vi "edit.vi"(8 "error in (no error)":errorcluster, 11 "BaseSetting in":refnum<class "ProcessSettings.lvclass">) -> (0 "error out":errorcluster, 2 "cancelIsTrue out":bool, 3 "BaseSetting out":refnum<class "ProcessSettings.lvclass">)   [LabVIEW 2016, in "Settings.lvlib" / "ProcessSettings.lvclass"]
uses:
  ProcessSettings.lvclass
  home/andres/ct_cmpuserevents/ComponentTemplateCore/Settings/Settings/Setting.lvclass
  ConfigurationTC/ConfigurationTypedefs/Base/SettingAliases.ctl
  ConfigurationTC/ConfigurationTypedefs/Base/SettingAlias.ctl
  ConfigurationTC/ConfigurationTypedefs/Base/RecommendedSettings.ctl
  ConfigurationTC/ConfigurationTypedefs/Base/HeartbeatConfig.ctl
  ConfigurationTC/ConfigurationTypedefs/Base/SALVisSettings.ctl
  MiddlewareSALThisComponent/ProgrammaticInitialization/evntsToSubscribeView.ctl
  MiddlewareSALThisComponent/ProgrammaticInitialization/tlmtryToSubscribeView.ctl
  MiddlewareSALThisComponent/ProgrammaticInitialization/cmdsToSubscribeDL.ctl
  Settings/Setting.lvclass/Setting.ctl
  <vilib>/Utility/xml.llb/Write to XML File(string).vi
  Settings/Setting.lvclass
  ConfigurationTC/ConfigurationTypedefs/ConfigurationTypedefs.lvlib
  MiddlewareSALThisComponent/ProgrammaticInitialization/ProgrammaticInitialization.lvclass
panel:
  in  "SettingTab":T1(tab)
  in  "Aliases":T2
  in  "GenericSALDefinitions":T4={"Subsystem"="EXA", "SAL Vis Path"=path "/home/andres/ts_cbp/ts_sallv_calibrationcbp/VIs", "Events"=["RejectedCommand", "SummaryState", "LoopTimeOutOfRange", "InternalCommand", "Heartbeat", "ErrorCode", "DetailedState", "AppliedSettingsMatchStart", "SettingVersions"], "Telemetry"=["Timestamp", "LoopTimems"], "Commands"=["Start", "Standby", "Enable", "Disable", "ExitControl"]}
  in  "RecommendedSettings":T8
  in  "heartbeatConfig":T9={"Heartbeat Interval (s)"=1.0, "Heartbeat Timeout (s)"=5.0} {"Heartbeat Timeout (s)" min=0.5 max=60.0 step=0.1 format="%.1f"; "Heartbeat Interval (s)" min=0.1 max=10.0 step=0.1 format="%.1f"}
  in  "cancelIsTrue":bool
  out "String":string
  in  "saveIsTrue":bool
  in  "Listbox":i32(listbox)
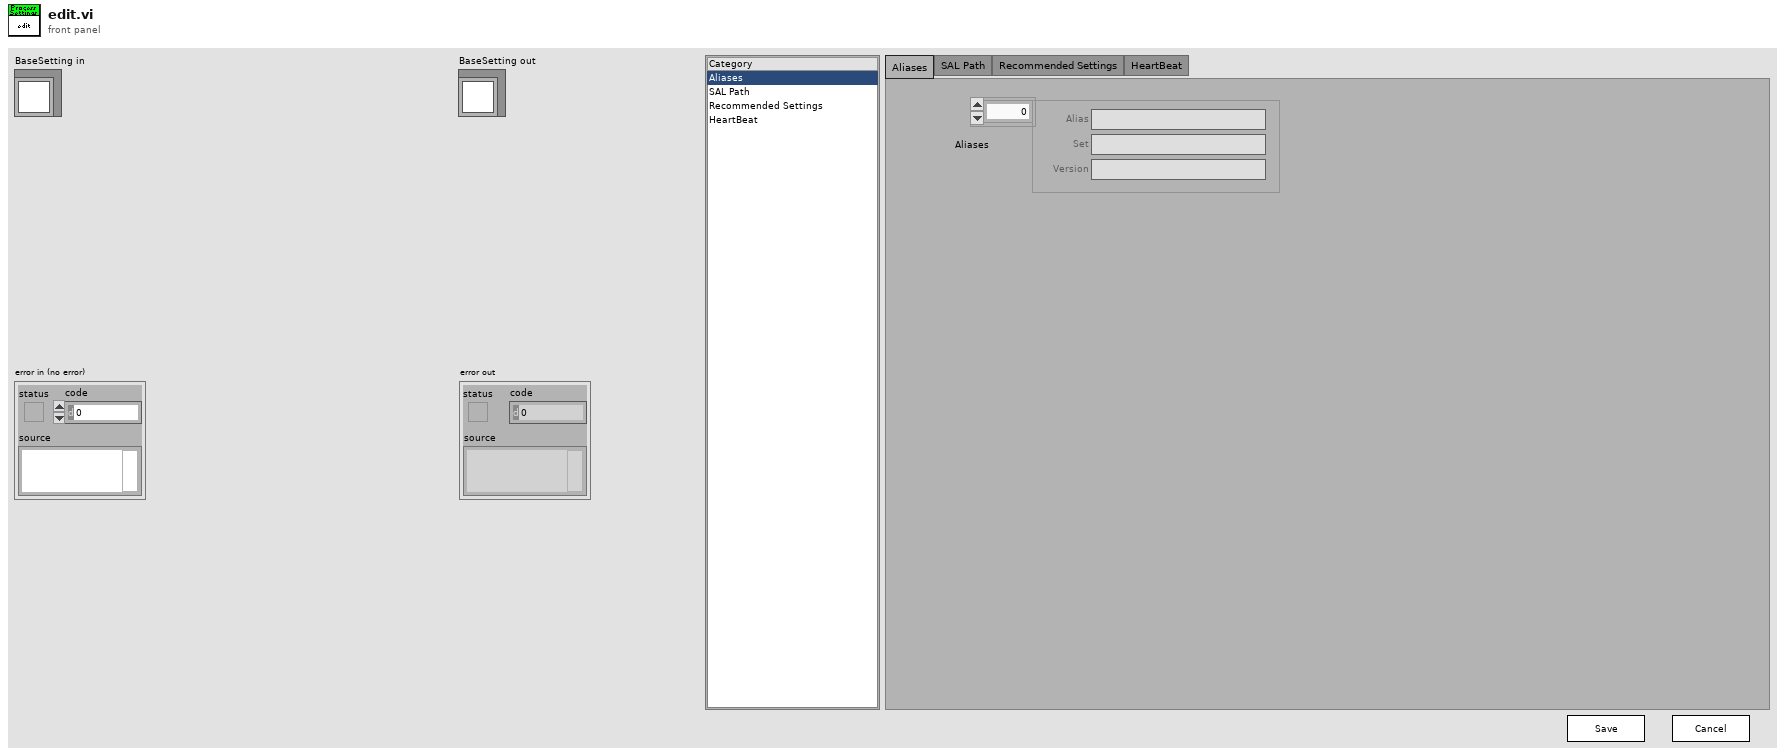
[diagram p1: front panel]
types:
  T1 = enum32{"Aliases", "SAL Path", "Recommended Settings", "HeartBeat"}
  T2 = typedef "ConfigurationTypedefs.lvlib/SettingAliases.ctl" = cluster{"Aliases":T3[]}
  T3 = typedef "ConfigurationTypedefs.lvlib/SettingAlias.ctl" = cluster{"Alias":string, "Set":string, "Version":string}
  T4 = typedef "ConfigurationTypedefs.lvlib/SALVisSettings.ctl" = cluster{"Subsystem":string, "SAL Vis Path":path, "Events":T5, "Telemetry":T6, "Commands":T7}
  T5 = typedef "ProgrammaticInitialization.lvclass/evntsToSubscribeView.ctl" = string[]
  T6 = typedef "ProgrammaticInitialization.lvclass/tlmtryToSubscribeView.ctl" = string[]
  T7 = typedef "ProgrammaticInitialization.lvclass/cmdsToSubscribeDL.ctl" = string[]
  T8 = typedef "ConfigurationTypedefs.lvlib/RecommendedSettings.ctl" = cluster{"RecommendedSetting\nVersions":string[], "RecommendedSettings\nLabels":string[]}
  T9 = typedef "ConfigurationTypedefs.lvlib/HeartbeatConfig.ctl" = cluster{"Heartbeat Interval (s)":dbl, "Heartbeat Timeout (s)":dbl}
  T10 = enum16{"open", "replace", "create", "open or create", "replace or create", "replace or create with confirmation"}
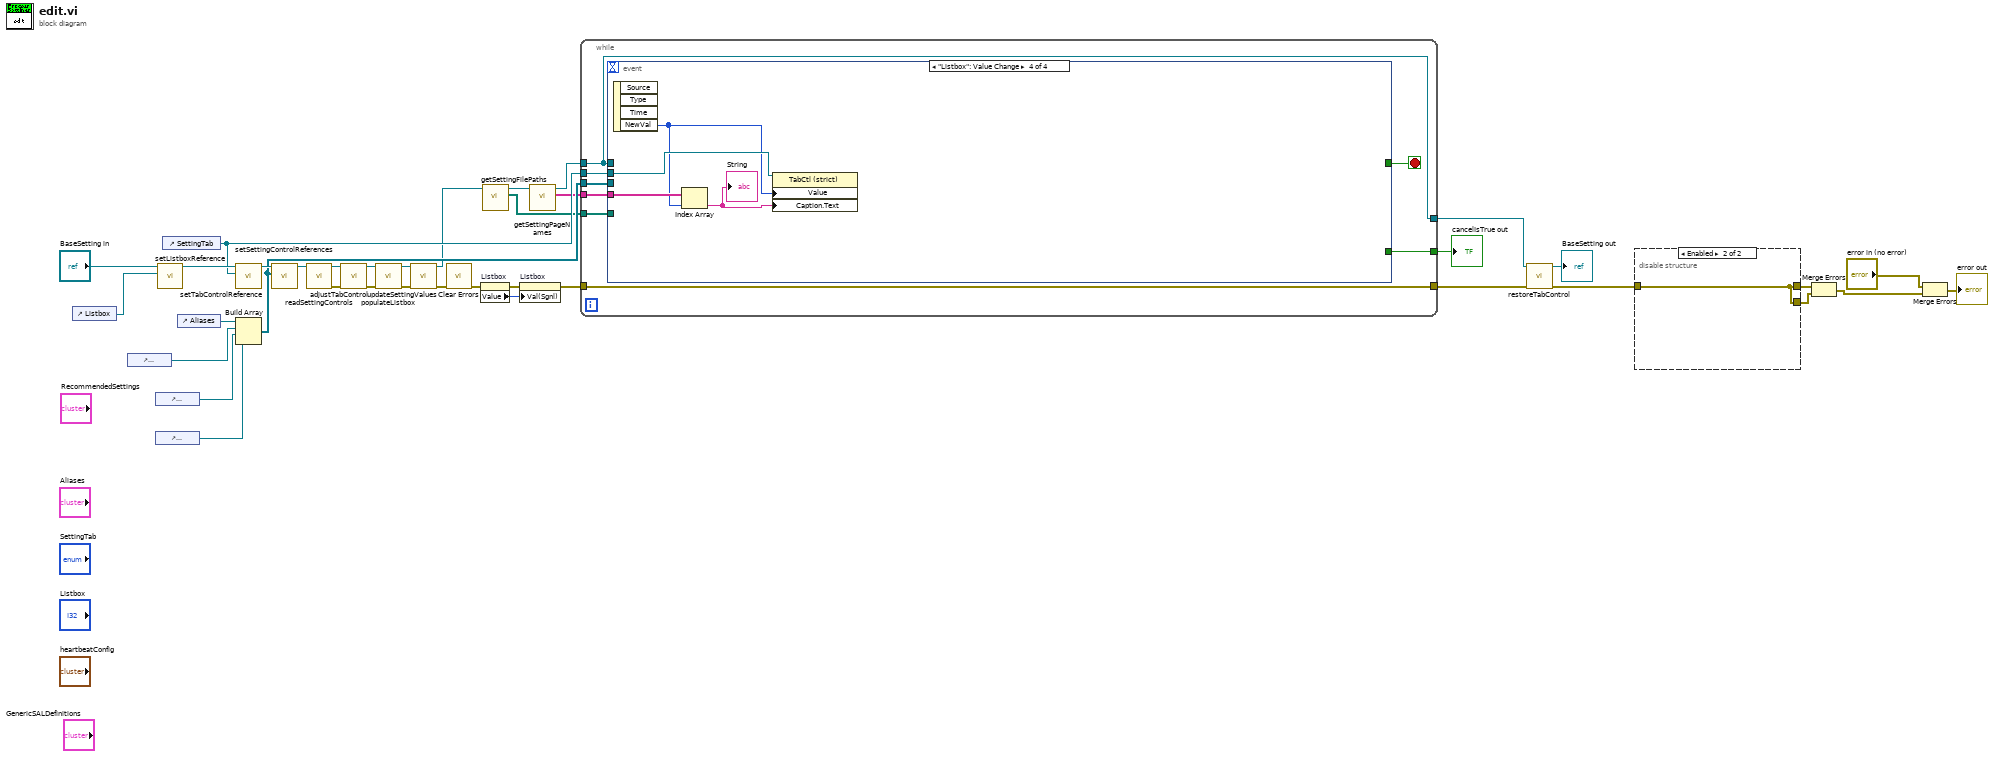
[diagram p0: block diagram]
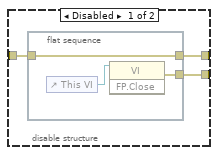
[diagram p2: hidden frame]
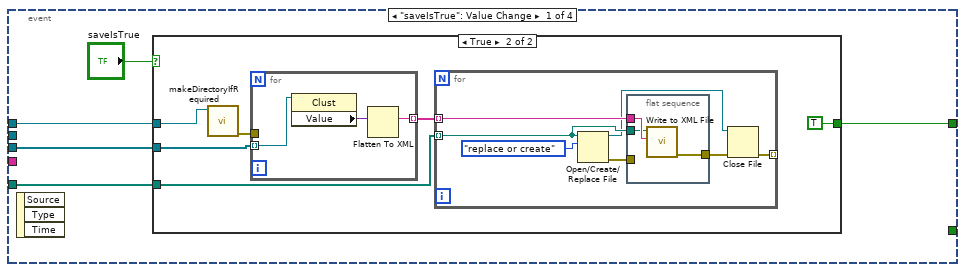
[diagram p3: hidden frame]
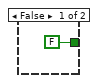
[diagram p4: hidden frame]
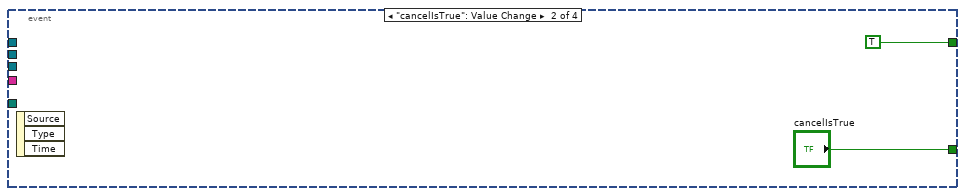
[diagram p5: hidden frame]
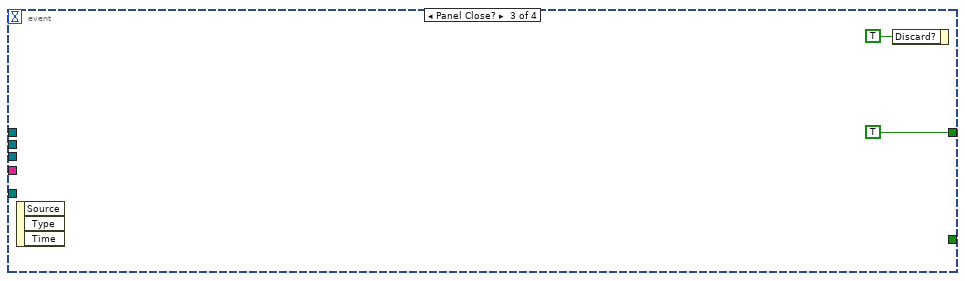
[diagram p6: hidden frame]
diagram:
  n1 = control-ref of="Listbox"() -> (w26:refnum<vi>)
  n2 = control-ref of="RecommendedSettings"() -> (w27:refnum<vi>)
  n3 = control-ref of="heartbeatConfig"() -> (w2:refnum<vi>)
  n4 = control-ref of="GenericSALDefinitions"() -> (w1:refnum<vi>)
  n5 = call "setListboxReference.vi"("ListboxReference"=w26, "Setting in"="BaseSetting in") -> ("Setting out"=w25:refnum<class "ProcessSettings.lvclass">)  [unwired: 9 in]
  n6 = control-ref of="SettingTab"() -> (w23:refnum<vi>)
  n7 = control-ref of="Aliases"() -> (w28:refnum<vi>)
  n8 = call "setTabControlReference.vi"("TabControlReference"=w23, "Setting in"=w25) -> ("Setting out"=w24:refnum<class "ProcessSettings.lvclass">)  [unwired: 9 in]
  n9 = Build Array(w28, w27, w2, w1) -> (w22:refnum<vi>[])
  n10 = call "setSettingControlReferences.vi"("SettingControlReferences"=w22, "Setting in"=w24) -> ("Setting out"=w17:refnum<class "ProcessSettings.lvclass">)  [unwired: 9 in]
  n11 = call "readSettingControls.vi"("BaseSetting in"=w17) -> ("error out"=w12:errorcluster, "BaseSetting out"=w16:refnum<class "ProcessSettings.lvclass">)  [unwired: 9 in]
  n12 = call "adjustTabControl.vi"("error in (no error)"=w12, "BaseSetting in"=w16) -> ("error out"=w11:errorcluster, "BaseSetting out"=w15:refnum<class "ProcessSettings.lvclass">)  [unwired: 8 in]
  n13 = call "populateListbox.vi"("error in (no error)"=w11, "BaseSetting in"=w15) -> ("error out"=w10:errorcluster, "BaseSetting out"=w14:refnum<class "ProcessSettings.lvclass">)  [unwired: 8 in]
  n14 = call "updateSettingValues.vi"("error in (no error)"=w10, "BaseSetting in"=w14) -> ("error out"=w4:errorcluster, "BaseSetting out"=w13:refnum<class "ProcessSettings.lvclass">)  [unwired: 8 in]
  n15 = call <vilib>:"Clear Errors.vi"("error in (no error)"=w4) -> ("error out"=w3:errorcluster)  [unwired: 5 in, 1 out]
  n16 = property on="Listbox" class="LstBox (strict)"(error in=w3) -> (error out=w36:errorcluster, "Value"=w37:i32)  [unwired: 1 in, 1 out]
  n17 = call "getSettingFilePaths.vi"("Setting in"=w13) -> ("SettingFilePaths"=w19:path[], "Setting out"=w21:refnum<class "ProcessSettings.lvclass">)  [unwired: 9 in]
  n18 = property on="Listbox" class="LstBox (strict)"(error in=w36, "Val(Sgnl)"=w37) -> (error out=w29:errorcluster)  [unwired: 1 in, 1 out]
  n19 = call "getSettingPageNames.vi"("Setting in"=w21) -> ("SettingPageNames"=w20:string[], "Setting out"=w18:refnum<class "ProcessSettings.lvclass">)  [unwired: 9 in]
  n20 = while {
    tunnel: w19 -> [w45]
    tunnel: w20 -> [w44]
    tunnel: w23 -> [w41]
    tunnel: w22 -> [w43]
    tunnel: [w38] -> w9
    tunnel: w18 -> [w38]
    tunnel: w29 -> [w40]
    tunnel: [w40] -> w6
    tunnel: [w39] -> w30
    stop <- w42 stop-if-true
    n21 = event shown="[3] \"Listbox\": Value Change" {
      selector: _ -> [_ _ _ _]
      dyn-events: _ -> [_ _ _ _]
      timeout: _ -> [_ _ _ _]
      tunnel: [w46 TRUE TRUE _] -> w42
      tunnel: w45 -> [w50 _ _ _]
      tunnel: w44 -> [_ _ _ w77]
      tunnel: w41 -> [_ _ _ w78]
      tunnel: w43 -> [w49 _ _ _]
      tunnel: [_ "cancelIsTrue" _ _] -> w39
      tunnel: w38 -> [w48 _ _ _]
      event "saveIsTrue": Value Change {
        n22 = event-data() -> ()  [unwired: 1 in, 3 out]
        n23 = case shown="True" "saveIsTrue" {
          tunnel: w50 -> [_ w57]
          tunnel: w49 -> [_ w56]
          tunnel: w48 -> [_ w53]
          tunnel: [FALSE TRUE] -> w46
          frame False {
          }
          frame True {
            n24 = call "makeDirectoryIfRequired.vi"("BaseSetting in"=w53) -> ("error out"=w52:errorcluster)  [unwired: 9 in, 1 out]
            n25 = for {
              tunnel: w56 -> [w70] mode=indexing
              tunnel: [w68] -> w55 mode=indexing
              tunnel: w52 -> [_]
              n26 = property class="Clust"(reference=w70) -> ("Value"=w69:variant)  [unwired: 1 in, 2 out]
              n27 = Flatten To XML(anything=w69) -> (xml string=w68:string)
            }
            n28 = for {
              tunnel: w57 -> [w61] mode=indexing
              tunnel: w55 -> [w64] mode=indexing
              tunnel: [w58] -> _ mode=indexing
              n29 = Open/Create/Replace File(file path (use dialog)=w61, operation (0:open)=T10."replace or create") -> (refnum out=w60:refnum<file>, error out=w62:errorcluster)  [unwired: 4 in, 1 out]
              n30 = flat-sequence {
                tunnel: w64 -> [w67]
                tunnel: [w66] -> w59
                tunnel: w62 -> [_]
                tunnel: w61 -> [w65]
                frame #0 {
                  n31 = call-poly <vilib>:"Write to XML File.vi"("XML Input"=w67, "XML File Path"=w65) -> ("error out"=w66:errorcluster)  [unwired: 7 in, 2 out]
                }
              }
              n32 = Close File(refnum=w60, error in=w59) -> (error out=w58:errorcluster)  [unwired: 1 out]
            }
          }
        }
      }
      event "cancelIsTrue": Value Change {
        n33 = event-data() -> ()  [unwired: 1 in, 3 out]
      }
      event Panel Close? {
        n34 = event-data() -> ()  [unwired: 1 in, 3 out]
        n35 = event-data("Discard?"=TRUE) -> ()  [unwired: 1 in, 1 out]
      }
      event "Listbox": Value Change {
        n36 = event-data() -> ("NewVal"=w76:i32)  [unwired: 1 in, 3 out]
        n37 = Index Array(array=w77, index=w76) -> (element=w75:string)
        "String" <- w75
        n38 = property class="TabCtl (strict)"(reference=w78, "Value"=w76, "Caption.Text"=w75) -> ()  [unwired: 1 in, 2 out]
      }
    }
  }
  "cancelIsTrue out" <- w30
  n39 = call "restoreTabControl.vi"("error in (no error)"=w6, "BaseSetting in"=w9) -> ("error out"=w7:errorcluster, "BaseSetting out"=→"BaseSetting out":refnum<class "ProcessSettings.lvclass">)  [unwired: 8 in]
  n40 = disable-structure shown="Enabled" {
    disable-tunnel: [w81 w85] -> w33
    disable-tunnel: [w80 w85] -> w31
    disable-tunnel: w7 -> [w79 w85]
    frame Disabled {
      n41 = flat-sequence {
        tunnel: [w83] -> w81
        tunnel: [w82] -> w80
        tunnel: w79 -> [w82]
        frame #0 {
          n42 = control-ref of="This VI"() -> (w84:refnum<vi>)
          n43 = invoke class="VI" method="FP.Close"(reference=w84) -> (error out=w83:errorcluster)  [unwired: 2 in, 2 out]
        }
      }
    }
    frame Enabled {
    }
  }
  n44 = Merge Errors(w31, w33) -> (w32:errorcluster)
  n45 = Merge Errors("error in (no error)", w32) -> (→"error out":errorcluster)
